vi "Probe orientation info.vi"(6 "az":sgl=1.0, 7 "ax_cal":sgl, 8 "ay":sgl, 9 "ax":sgl, 10 "az_cal":sgl=1.0, 11 "ay_cal":sgl) -> (0 "Relative roll (deg)":sgl, 1 "Calib. pitch (deg)":sgl, 2 "Calib. roll (deg)":sgl, 3 "Pitch (deg)":sgl, 4 "Relative pitch (deg)":sgl, 5 "Roll (deg)":sgl)   [LabVIEW 2018]
panel:
  # "PN 23/03/18"
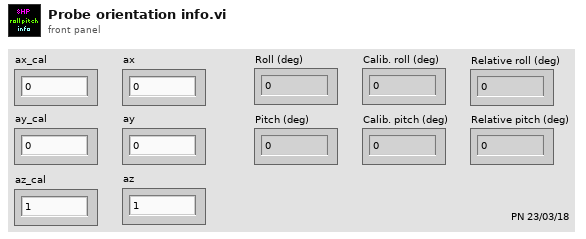
[diagram p1: front panel]
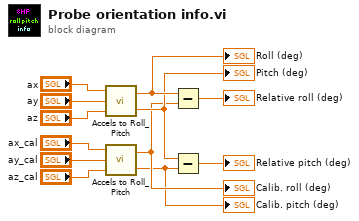
[diagram p0: block diagram]
diagram:
  n1 = call "Accels to Roll_Pitch.vi"("az"="az", "ay"="ay", "ax"="ax") -> ("Pitch (deg)"=w3:sgl, "Roll (deg)"=w4:sgl)
  "Roll (deg)" <- w4
  "Pitch (deg)" <- w3
  n2 = call "Accels to Roll_Pitch.vi"("az"="az_cal", "ay"="ay_cal", "ax"="ax_cal") -> ("Pitch (deg)"=w1:sgl, "Roll (deg)"=w2:sgl)
  "Calib. roll (deg)" <- w2
  "Calib. pitch (deg)" <- w1
  n3 = Subtract(x=w4, y=w2) -> (x-y=→"Relative roll (deg)":sgl)
  n4 = Subtract(x=w3, y=w1) -> (x-y=→"Relative pitch (deg)":sgl)
